vi "ExplorerTree Example.vi"() -> ()   [LabVIEW 2015]
doc: "This example gets the content of a folder and displays it in a tree control. Similar to file explorer windows, this sorts alphabetically by sub-directories then files. The file extension icons are returned as a custom symbols array to be referenced in the tree control. If a file icon is not found, this queries the operating system shell icon and keeps the glyph cached.\n\nCreated By: Ryan Pacini"
panel:
  in  "Folder Path":path
  in  "Tree":string(tree)
  # "Instructions: Select folder path then press run"
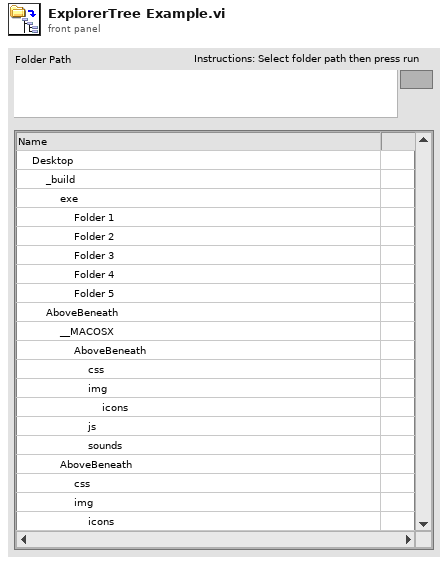
[diagram p1: front panel]
types:
  T1 = typedef "imagedata.ctl" = cluster{"image type":i32, "image depth":i32, "image":u8[], "mask":u8[], "colors":u32[], "Rectangle":cluster{"left":i16, "top":i16, "right":i16, "bottom":i16}}
  T2 = cluster{"Left Cell String":string, "Child Text":string[], "Child Tag":string, "Item Indent":i32, "Child Only?":bool, "Glyph Index":i32}[]
  T3 = cluster{"Left Cell String":string, "Child Text":string[], "Child Tag":string, "Item Indent":i32, "Child Only?":bool, "Glyph Index":i32}
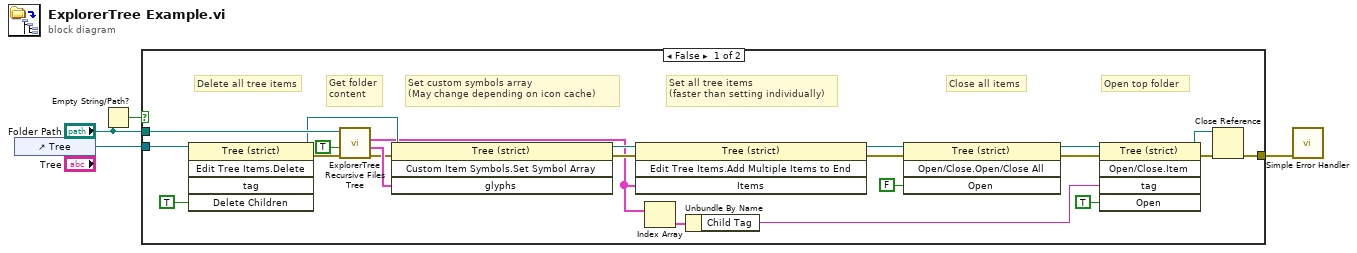
[diagram p0: block diagram]
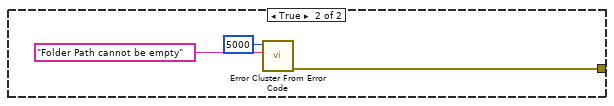
[diagram p2: hidden frame]
diagram:
  n1 = control-ref of="Tree"() -> (w4:refnum<vi>)
  n2 = Empty String/Path?(string/path="Folder Path") -> (empty?=w1:bool)
  n3 = case shown="False" w1 {
    tunnel: w4 -> [w26 _]
    tunnel: "Folder Path" -> [w23 _]
    tunnel: [w7 w27] -> w3
    frame False {
      # "Open top folder"
      # "Close all items"
      # "Set all tree items\n(faster than setting individually)"
      # "Set custom symbols array\n(May change depending on icon cache)"
      # "Get folder\ncontent"
      # "Delete all tree items"
      n4 = invoke class="Tree (strict)" method="Edit Tree Items.Delete"(reference=w26, "Delete Children"=TRUE ("Delete Children?")) -> (reference out=w22:refnum<vi>, error out=w24:errorcluster)  [unwired: 3 in, 3 out]
      n5 = call "ExplorerTree Recursive Files Tree.vi"("error in (no error)"=w24, "Continue Recursing on Error? (F)"=TRUE, "Folder Path"=w23) -> ("error out"=w6:errorcluster, "Glyphs"=w21:T1[], "Items"=w13:T2)  [unwired: 5 in, 1 out]
      n6 = invoke class="Tree (strict)" method="Custom Item Symbols.Set Symbol Array"(reference=w22, error in=w6, "glyphs"=w21) -> (reference out=w19:refnum<vi>, error out=w20:errorcluster)  [unwired: 1 in, 2 out]
      n7 = invoke class="Tree (strict)" method="Edit Tree Items.Add Multiple Items to End"(reference=w19, error in=w20, "Items"=w13) -> (reference out=w17:refnum<vi>, error out=w18:errorcluster)  [unwired: 1 in, 2 out]
      n8 = Index Array(array=w13) -> (element=w12:T3)  [unwired: 1 in]
      n9 = Unbundle By Name(w12) -> ("Child Tag"=w11:string)
      n10 = invoke class="Tree (strict)" method="Open/Close.Open/Close All"(reference=w17, error in=w18, "Open"=FALSE ("Open?")) -> (reference out=w15:refnum<vi>, error out=w14:errorcluster)  [unwired: 1 in, 2 out]
      n11 = invoke class="Tree (strict)" method="Open/Close.Item"(reference=w15, error in=w14, "tag"=w11, "Open"=TRUE ("Open?")) -> (reference out=w8:refnum<vi>, error out=w9:errorcluster)  [unwired: 1 in, 3 out]
      n12 = Close Reference(reference=w8, error in (no error)=w9) -> (error out=w7:errorcluster)
    }
    frame True {
      n13 = call <vilib>:"Error Cluster From Error Code.vi"("error message (\"\")"="Folder Path cannot be empty" ("source"), "error code (0)"=5000) -> ("error out"=w27:errorcluster)  [unwired: 7 in]
    }
  }
  n14 = call <vilib>:"Simple Error Handler.vi"("error in (no error)"=w3) -> ()  [unwired: 4 in, 5 out]
